vi "FlexDDS-NG_DCP_StartStop.vi"(9 "start (T) stop (F)":bool=TRUE, 10 "Channels":T1(ring)=enum."Both channels", 11 "initial instruction string":string) -> (3 "appended instruction string":string="dcp start\r")   [LabVIEW 2016]
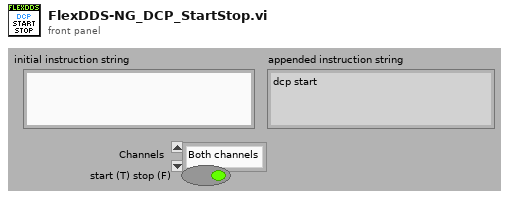
[diagram p1: front panel]
types:
  T1 = enum32{"Channel 0", "Channel 1", "Both channels"}
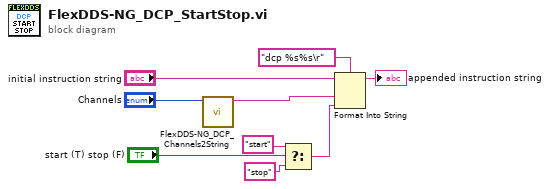
[diagram p0: block diagram]
diagram:
  n1 = call "FlexDDS-NG_DCP_Channels2String.vi"("Channels"="Channels") -> ("channels string"=w2:string)  [unwired: 10 in]
  n2 = Select(t="start" ("format string"), s="start (T) stop (F)", f="stop" ("format string")) -> (s? t:f=w1:string)
  n3 = Format Into String(format string="dcp %s%s\r", initial string="initial instruction string", w2, w1) -> (resulting string=→"appended instruction string":string)  [unwired: 1 in, 1 out]
